vi "Pasco Turning Logic.vi"(11 "Delta Angle":dbl) -> (1 "Case Selector":bool, 3 "Corrected Angle":dbl)   [LabVIEW 2011]
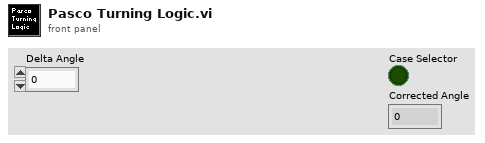
[diagram p1: front panel]
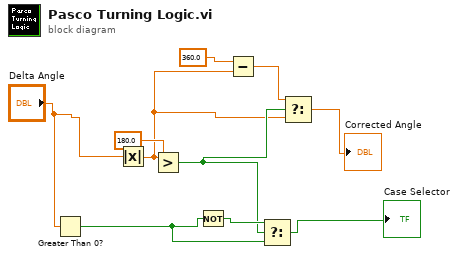
[diagram p0: block diagram]
diagram:
  n1 = Greater Than 0?(x="Delta Angle") -> (x > 0?=w9:bool)
  n2 = Absolute Value(x="Delta Angle") -> (abs(x)=w1:dbl)
  n3 = Greater?(x=w1, y=180.0) -> (0:w5:bool)
  n4 = Not(x=w9) -> (.not. x?=w8:bool)
  n5 = Subtract(x=360.0, y=w1) -> (x-y=w4:dbl)
  n6 = Select(t=w8, s=w5, f=w9) -> (s? t:f=→"Case Selector":bool)
  n7 = Select(t=w4, s=w5, f=w1) -> (s? t:f=→"Corrected Angle":dbl)
